vi "Get VI Bookmarks.vi"(8 "error in (no error)":errorcluster, 11 "VI in":refnum<vi>) -> (0 "error out":errorcluster, 3 "BookmarkInfo":T1)   [LabVIEW 2023, in "VIDoc Parsing.lvlib"]
uses:
  VIDoc Parsing.lvlib
  <vilib>/Utility/miscctls.llb/LVBookmarkInfoTypeDef.ctl
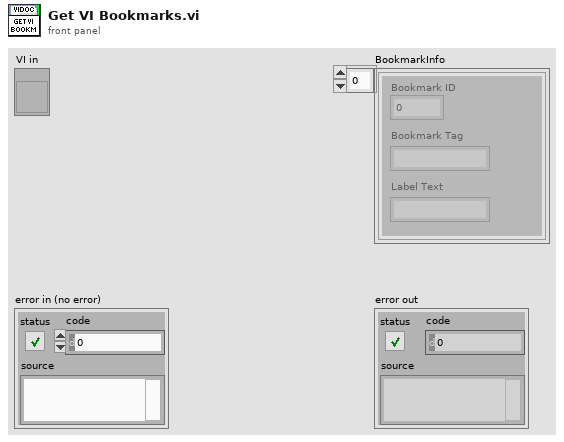
[diagram p1: front panel]
types:
  T1 = typedef "LVBookmarkInfoTypeDef.ctl" = cluster{"Bookmark ID":u32, "Bookmark Tag":string, "Label Text":string}[]
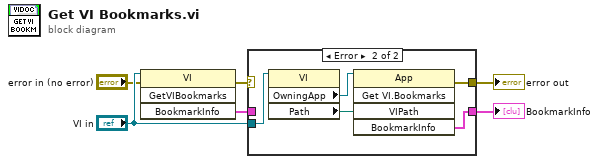
[diagram p0: block diagram]
diagram:
  n1 = invoke class="VI" method="GetVIBookmarks"(reference="VI in", error in="error in (no error)") -> (error out=w1:errorcluster, "BookmarkInfo"=w2:T1)  [unwired: 2 in, 2 out]
  n2 = case shown="Error" w1 {
    selector: w1 -> [w7 _]
    tunnel: w2 -> [w8 _]
    tunnel: [w8 w12] -> w4
    tunnel: [w7 w13] -> w5
    tunnel: "VI in" -> [_ w11]
    frame No Error {
    }
    frame Error {
      n3 = property class="VI"(reference=w11) -> ("OwningApp"=w9:refnum<vi>, "Path"=w10:path)  [unwired: 1 in, 2 out]
      n4 = invoke class="App" method="Get VI.Bookmarks"(reference=w9, "VIPath"=w10) -> (error out=w13:errorcluster, "BookmarkInfo"=w12:T1)  [unwired: 3 in, 3 out]
    }
  }
  "error out" <- w5
  "BookmarkInfo" <- w4
